vi "CreateListener.vi"(0 "Socket Listener in":refnum<class "Socket Communication.lvclass">, 5 "error in (no error)":errorcluster) -> (14 "Socket Listener out":refnum<class "Socket Communication.lvclass">, 19 "error out":errorcluster)   [LabVIEW 2016, in "Socket Communication.lvclass"]
uses:
  Socket Communication.lvclass
  Socket Communication.lvclass/Socket Communication.ctl
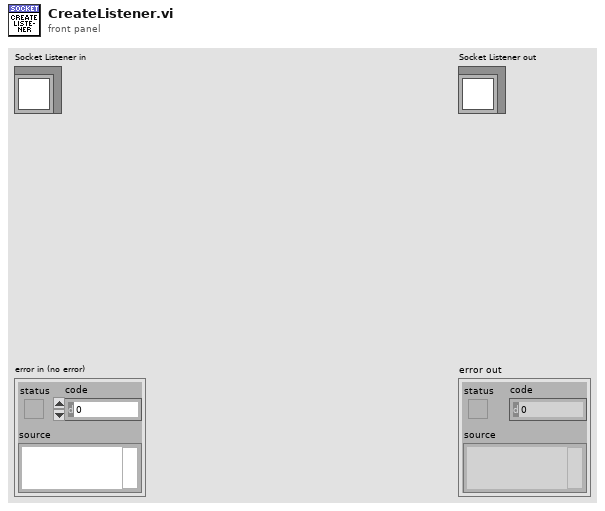
[diagram p1: front panel]
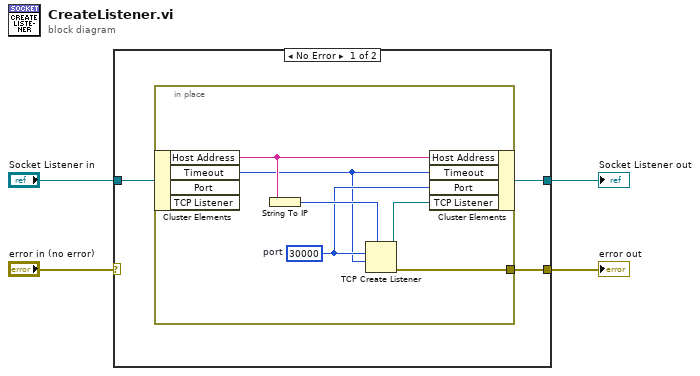
[diagram p0: block diagram]
diagram:
  n1 = case shown="No Error" "error in (no error)" {
    selector: "error in (no error)" -> [_ w15]
    tunnel: [w7 w15] -> w3
    tunnel: [w5 w14] -> w1
    tunnel: "Socket Listener in" -> [w6 w14]
    frame No Error {
      n2 = in-place {
        in-place-border: [w13] -> w7
        w10 = u16 30000  # port
        n3 = in-place-cluster #1(w6) -> ("Host Address"=w9:string, "Timeout"=w8:i32)  [unwired: 2 out]
        n4 = String To IP(1:w9) -> (0:w12:u32)
        n5 = TCP Create Listener(7:w12, 9:w8, 10:w10) -> (0:w13:errorcluster, 3:w11:refnum<k5>)  [unwired: 2 in, 1 out]
        n6 = in-place-cluster #1("Host Address"=w9, "Timeout"=w8, "Port"=w10, "TCP Listener"=w11) -> (w5:refnum<class "Socket Communication.lvclass">)
      }
    }
    frame Error {
    }
  }
  "error out" <- w3
  "Socket Listener out" <- w1
